vi "Facade.vi"(0 "Data In":T4, 2 "Display State In":T2, 3 "Container State":T3) -> (6 "Data Out":T4, 7 "Display State Out":T2, 8 "Action":T1)   [LabVIEW 2010, in "magic ring.xctl"]
uses:
  magic ring.xctl
  controls/Data.ctl
  <vilib>/_xctls/Container State.ctl
  controls/State.ctl
  <vilib>/_xctls/Action.ctl
  <vilib>/_xctls/XControlSupport.lvlib
panel:
  in  "List":i32(listbox)
  in  "string":string
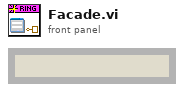
[diagram p1: front panel]
types:
  T1 = typedef "XControlSupport.lvlib/Action.ctl" = cluster{"Data Changed?":bool, "State Changed?":bool, "Action Name":string}
  T2 = typedef "magic ring.xctl/State.ctl" = cluster{"item list":string[], "displayed items":string[], "max rows (5)":i32, "min rows (2)":i32, "selection":i32}
  T3 = typedef "XControlSupport.lvlib/Container State.ctl" = cluster{"Indicator?":bool, "Run Mode?":bool, " Refnum":refnum<vi>}
  T4 = typedef "magic ring.xctl/Data.ctl" = string
  T5 = enum8{"Enabled", "Disabled", "Disabled and Grayed Out"}
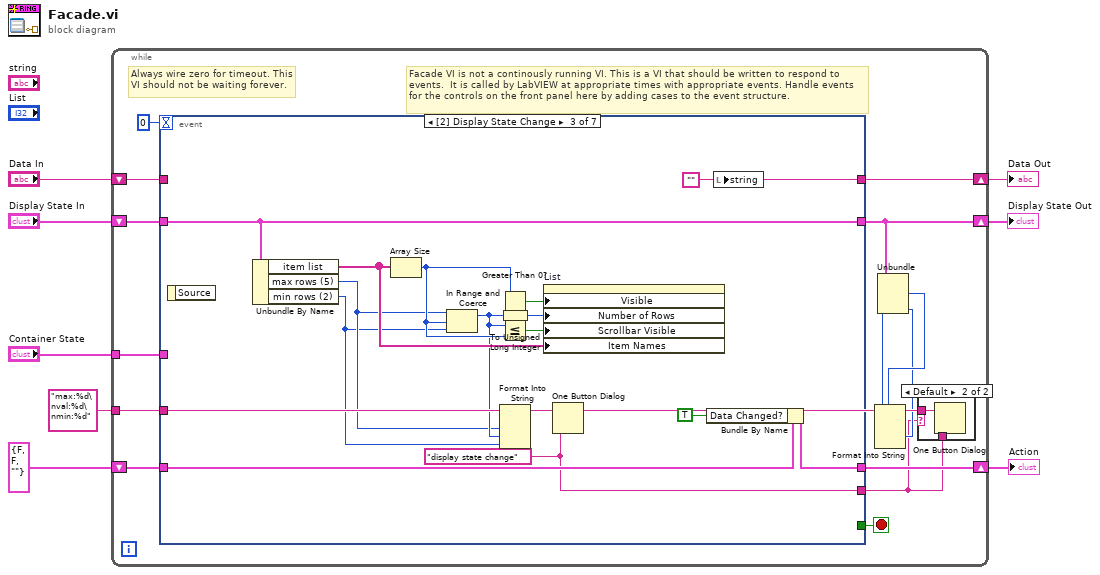
[diagram p0: block diagram]
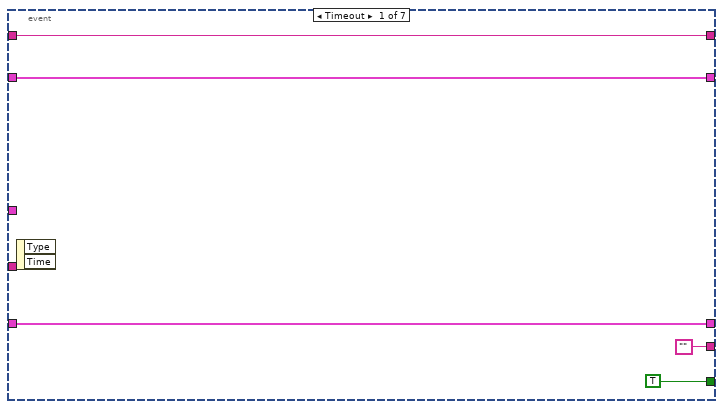
[diagram p3: hidden frame]
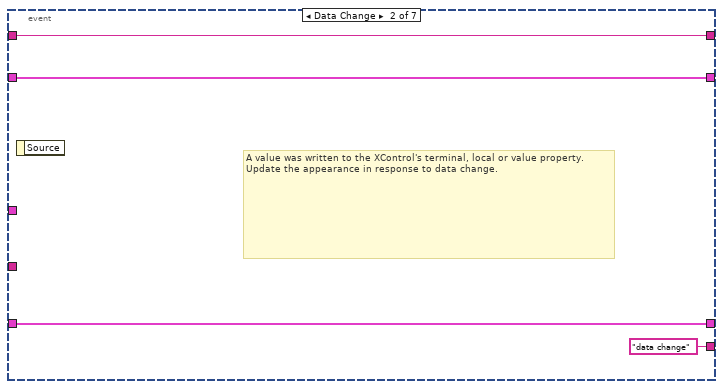
[diagram p4: hidden frame]
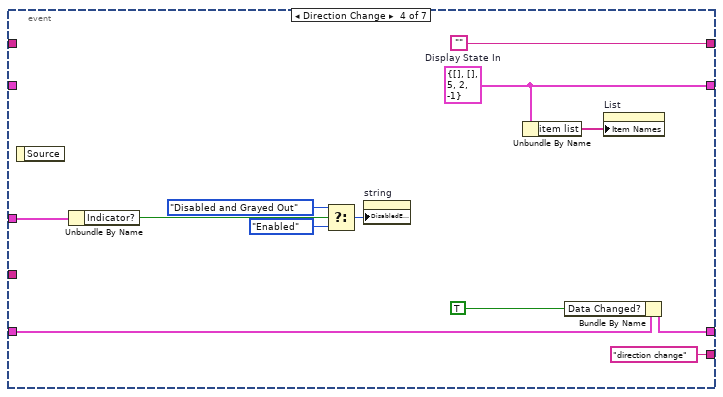
[diagram p5: hidden frame]
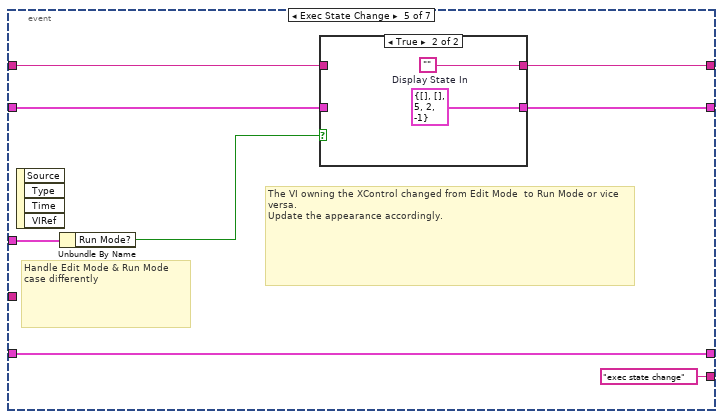
[diagram p6: hidden frame]
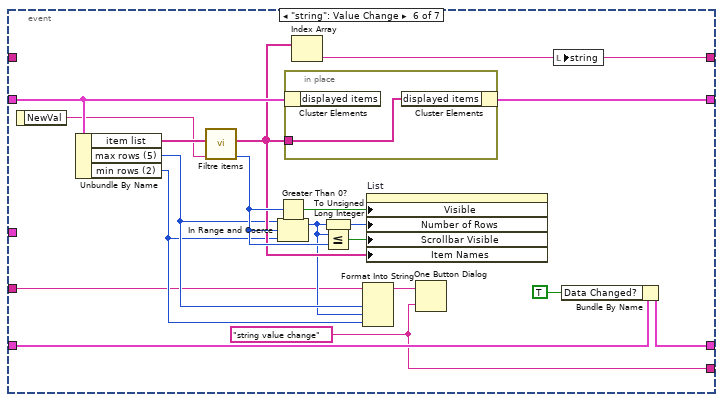
[diagram p8: hidden frame]
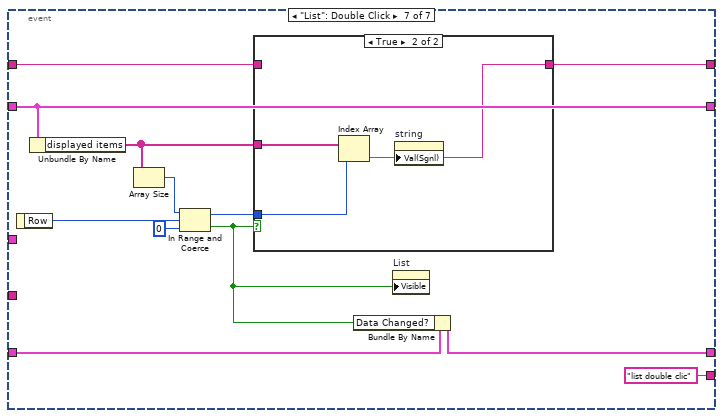
[diagram p9: hidden frame]
diagram:
  n1 = while {
    shift-right: [w13] -> w5
    shift-left: "Display State In" -> [w23]
    tunnel: "Container State" -> [w20]
    shift-right: [w18] -> w8
    shift-left: "Data In" -> [w19]
    shift-right: [w16] -> w3
    shift-left: T1 {"Data Changed?"=FALSE, "State Changed?"=FALSE, "Action Name"=""} ("Action") -> [w17]
    tunnel: "max:%d\nval:%d\nmin:%d" -> [w14]
    stop <- w22 stop-if-true
    # "Facade VI is not a continously running VI. This is a VI that should be written to respond to events.  It is called by LabVIEW at appropriate times with appropriate events. Handle events for the controls on the front panel here by adding cases to the event structure."
    # "Always wire zero for timeout. This\nVI should not be waiting forever."
    n2 = event shown="[2] Display State Change" {
      selector: _ -> [_ _ _ _ _ _ _]
      dyn-events: _ -> [_ _ _ _ _ _ _]
      timeout: 0 -> [_ _ _ _ _ _ _]
      tunnel: w23 -> [w27 w34 w46 _ w65 w85 w99]
      tunnel: [w27 w34 w46 w53 w68 w83 w99] -> w13
      tunnel: [TRUE _ _ _ _ _ _] -> w22
      tunnel: w20 -> [_ _ _ w62 w70 _ _]
      tunnel: w19 -> [w28 w32 _ _ w64 _ w104]
      tunnel: [w28 w32 w45 "" w69 w81 w106] -> w18
      tunnel: [w29 w33 w42 w55 w66 w92 w97] -> w16
      tunnel: w17 -> [w29 w33 w43 w56 w66 w93 w98]
      tunnel: w14 -> [_ _ w36 _ _ w76 _]
      tunnel: ["" "data change" w35 "direction change" "exec state change" w75 "list double clic"] -> w9
      event Timeout {
        n3 = event-data() -> ()  [unwired: 1 in, 2 out]
      }
      event Data Change {
        # "A value was written to the XControl's terminal, local or value property.\nUpdate the appearance in response to data change."
        n4 = event-data() -> ()  [unwired: 1 in, 1 out]
      }
      event Display State Change {
        w35 = "display state change"
        w45 = ""
        n5 = event-data() -> ()  [unwired: 1 in, 1 out]
        n6 = Unbundle By Name(w46) -> ("item list"=w44:string[], "max rows (5)"=w38:i32, "min rows (2)"=w37:i32)
        n7 = Array Size(array=w44) -> (size(s)=w41:i32)
        n8 = In Range and Coerce(upper limit=w38, x=w41, lower limit=w37) -> (coerced(x)=w39:i32)  [unwired: 1 out]
        n9 = Greater Than 0?(x=w41) -> (x > 0?=w49:bool)
        n10 = To Unsigned Long Integer(number=w39) -> (unsigned 32bit integer=w48:u32)
        n11 = Less Or Equal?(x=w39, y=w41) -> (x <= y?=w47:bool)
        n12 = Format Into String(format string=w36, w38, w39, w37) -> (resulting string=w40:string)  [unwired: 2 in, 1 out]
        n13 = property on="List" class="ListBox (strict)"("Visible"=w49, "Number of Rows"=w48, "Scrollbar Visible"=w47, "Item Names"=w44) -> ()  [unwired: 2 in, 2 out]
        n14 = One Button Dialog(message=w40, button name ("OK")=w35) -> ()  [unwired: 1 out]
        n15 = Bundle By Name(cluster=w43, "Data Changed?"=TRUE) -> (w42:T1)
        n16 = local write "string"(w45) -> ()
      }
      event Direction Change {
        w53 = T2 {"item list"=[], "displayed items"=[], "max rows (5)"=5, "min rows (2)"=2, "selection"=-1}  # Display State In
        n17 = event-data() -> ()  [unwired: 1 in, 1 out]
        n18 = Unbundle By Name(w62) -> ("Indicator?"=w61:bool)
        n19 = Select(t=T5."Disabled and Grayed Out", s=w61, f=T5."Enabled") -> (s? t:f=w58:T5)
        n20 = property on="string" class="Str"("DisabledEnum"=w58) -> ()  [unwired: 2 in, 2 out]
        n21 = Unbundle By Name(w53) -> ("item list"=w52:string[])
        n22 = Bundle By Name(cluster=w56, "Data Changed?"=TRUE) -> (w55:T1)
        n23 = property on="List" class="LstBox (strict)"("Item Names"=w52) -> ()  [unwired: 2 in, 2 out]
      }
      event Exec State Change {
        # "The VI owning the XControl changed from Edit Mode  to Run Mode or vice versa.\nUpdate the appearance accordingly."
        # "Handle Edit Mode & Run Mode\ncase differently"
        n24 = event-data() -> ()  [unwired: 1 in, 4 out]
        n25 = Unbundle By Name(w70) -> ("Run Mode?"=w67:bool)
        n26 = case shown="True" w67 {
          tunnel: [w71 ""] -> w69
          tunnel: [w72 w73] -> w68
          tunnel: w65 -> [w72 _]
          tunnel: w64 -> [w71 _]
          frame False {
          }
          frame True {
            w73 = T2 {"item list"=[], "displayed items"=[], "max rows (5)"=5, "min rows (2)"=2, "selection"=-1}  # Display State In
          }
        }
      }
      event "string": Value Change {
        w75 = "string value change"
        n27 = event-data() -> ("NewVal"=w84:string)  [unwired: 1 in]
        n28 = Unbundle By Name(w85) -> ("item list"=w90:string[], "max rows (5)"=w79:i32, "min rows (2)"=w78:i32)
        n29 = call "Filtre items.vi"("filtre"=w84, "item list"=w90) -> ("# match"=w86:i32, "filtred list"=w82:string[])  [unwired: 6 in]
        n30 = Greater Than 0?(x=w86) -> (x > 0?=w89:bool)
        n31 = In Range and Coerce(upper limit=w79, x=w86, lower limit=w78) -> (coerced(x)=w77:i32)  [unwired: 1 out]
        n32 = in-place {
          in-place-border: w82 -> [w94]
          n33 = in-place-cluster #1(w85) -> ()  [unwired: 1 out]
          n34 = in-place-cluster #1("displayed items"=w94) -> (w83:T2)
        }
        n35 = Index Array(array=w82) -> (element=w81:string)  [unwired: 1 in]
        n36 = To Unsigned Long Integer(number=w77) -> (unsigned 32bit integer=w88:u32)
        n37 = Less Or Equal?(x=w77, y=w86) -> (x <= y?=w87:bool)
        n38 = Format Into String(format string=w76, w79, w77, w78) -> (resulting string=w80:string)  [unwired: 2 in, 1 out]
        n39 = property on="List" class="ListBox (strict)"("Visible"=w89, "Number of Rows"=w88, "Scrollbar Visible"=w87, "Item Names"=w82) -> ()  [unwired: 2 in, 2 out]
        n40 = One Button Dialog(message=w80, button name ("OK")=w75) -> ()  [unwired: 1 out]
        n41 = local write "string"(w81) -> ()
        n42 = Bundle By Name(cluster=w93, "Data Changed?"=TRUE) -> (w92:T1)
      }
      event "List": Double Click {
        n43 = event-data() -> ("Row"=w105:i32)  [unwired: 1 in]
        n44 = Unbundle By Name(w99) -> ("displayed items"=w100:string[])
        n45 = Array Size(array=w100) -> (size(s)=w101:i32)
        n46 = In Range and Coerce(upper limit=w101, x=w105, lower limit=0) -> (coerced(x)=w102:i32, In Range?=w96:bool)
        n47 = case shown="True" w96 {
          tunnel: [w107 w108] -> w106
          tunnel: w104 -> [w107 _]
          tunnel: w102 -> [_ w109]
          tunnel: w100 -> [_ w110]
          frame False {
          }
          frame True {
            n48 = Index Array(array=w110, index=w109) -> (element=w108:string)
            n49 = property on="string" class="Str"("Val(Sgnl)"=w108) -> ()  [unwired: 2 in, 2 out]
          }
        }
        n50 = Bundle By Name(cluster=w98, "Data Changed?"=w96) -> (w97:T1)
        n51 = property on="List" class="LstBox (strict)"("Visible"=w96) -> ()  [unwired: 2 in, 2 out]
      }
    }
    n52 = Unbundle(w13) -> ("max rows (5)"=w12:i32, "min rows (2)"=w11:i32, "selection"=w10:i32)  [unwired: 2 out]
    n53 = Format Into String(format string=w14, w12, w10, w11) -> (resulting string=w15:string)  [unwired: 2 in, 1 out]
    n54 = case shown="Default" w9 {
      tunnel: w15 -> [_ w25]
      tunnel: w9 -> [_ w24]
      frame "\u0000" {
      }
      frame Default {
        n55 = One Button Dialog(message=w25, button name ("OK")=w24) -> ()  [unwired: 1 out]
      }
    }
  }
  "Display State Out" <- w5
  "Data Out" <- w8
  "Action" <- w3
